vi "HiFiveUnmatched_ComputePower.vi"(8 "Configurations":T1[](array[typedef]), 11 "Current Waveforms":waveform(dbl)[](array[waveform])) -> (3 "Power":waveform(dbl)[](array[waveform]))   [LabVIEW 2020]
uses:
  HiFiveUnmatched_PowerLineCfg.ctl
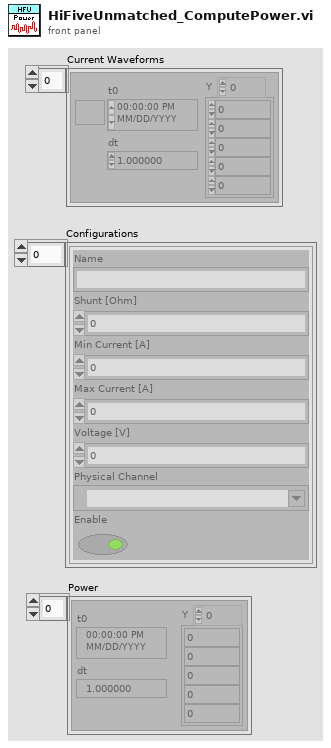
[diagram p1: front panel]
types:
  T1 = typedef "HiFiveUnmatched_PowerLineCfg.ctl" = cluster{"Name":string, "Shunt [Ohm]":dbl, "Min Current [A]":dbl, "Max Current [A]":dbl, "Voltage [V]":dbl, "Physical Channel":tag, "Enable":bool}
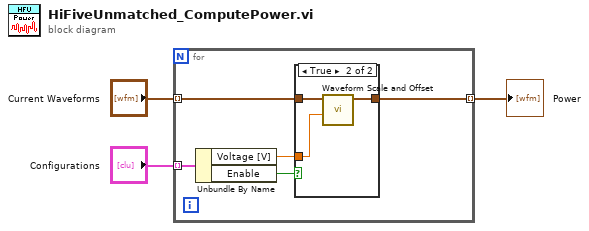
[diagram p0: block diagram]
diagram:
  n1 = for {
    tunnel: "Current Waveforms" -> [w5] mode=indexing
    tunnel: "Configurations" -> [w8] mode=indexing
    tunnel: [w4] -> w2 mode=indexing
    n2 = Unbundle By Name(w8) -> ("Voltage [V]"=w6:dbl, "Enable"=w7:bool)
    n3 = case shown="True" w7 {
      tunnel: w6 -> [_ w11]
      tunnel: w5 -> [w9 w12]
      tunnel: [w9 w10] -> w4
      frame False {
      }
      frame True {
        n4 = call <vilib>:"Waveform Scale and Offset.vi"("scale"=w11, "waveform in"=w12) -> ("waveform out"=w10:waveform(dbl))  [unwired: 8 in, 1 out]
      }
    }
  }
  "Power" <- w2
